vi "WM Limit Settings.vi"(1 "Limit Settings":T1={"Min Wave Period"=0.9, "Max Wave Period"=3.5, "Cutoff Frequency"=2.0, "Max 1/2 Piston Stroke"=0.16, "Max H/L"=0.07, "Max H/d"=0.65} {"Max H/d" format="%.2f"; "Max H/L" format="%.2f"; "Max 1/2 Piston Stroke" format="%.2f"; "Cutoff Frequency" format="%.2f"; "Max Wave Period" format="%.2f"; "Min Wave Period" format="%.2f"}) -> (0 "Limit Settings Output":T1 {"Max H/d" format="%.2f"; "Max H/L" format="%.2f"; "Max 1/2 Piston Stroke" format="%.2f"; "Cutoff Frequency" format="%.2f"; "Max Wave Period" format="%.2f"; "Min Wave Period" format="%.2f"})   [LabVIEW 2012]
panel:
  in  "OK":bool
  # "m"
  # "s"
  # "s"
  # "Hz"
  # "m"
  # "s"
  # "s"
  # "Hz"
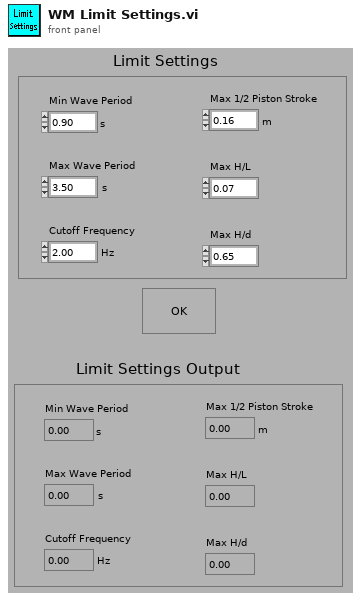
[diagram p1: front panel]
types:
  T1 = cluster{"Min Wave Period":dbl, "Max Wave Period":dbl, "Cutoff Frequency":dbl, "Max 1/2 Piston Stroke":dbl, "Max H/L":dbl, "Max H/d":dbl}
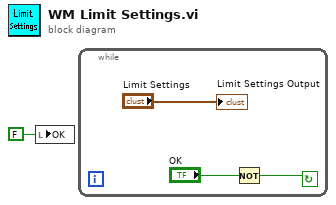
[diagram p0: block diagram]
diagram:
  n1 = local write "OK"(FALSE ("OK")) -> ()
  n2 = while {
    stop <- w3 continue-if-true
    n3 = Not(x="OK") -> (.not. x?=w3:bool)
    "Limit Settings Output" <- "Limit Settings"
  }
